vi "_FPGA_Truncation_U32_to_UFXP15.vi"(10 "U32_in":u32) -> (2 "FXP_+_15_15_out":fxp<+,15,15>)   [LabVIEW 2018]
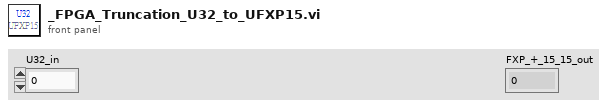
[diagram p1: front panel]
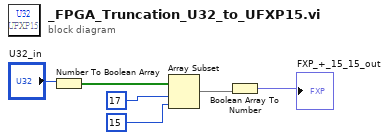
[diagram p0: block diagram]
diagram:
  n1 = Number To Boolean Array(number="U32_in") -> (Boolean array=w5:bool[])
  n2 = Array Subset(array=w5, index=17, length=15) -> (w2:bool[])
  n3 = Boolean Array To Number(Boolean array=w2) -> (number=→"FXP_+_15_15_out":fxp<+,15,15>)
